vi "Get settings chain.vi"(8 "error in (no error)":errorcluster, 11 "focusBase in":refnum<class "focus.lvclass">) -> (0 "error out":errorcluster, 1 "class name":string[](array[string]), 2 "settings":variant[](array[variant]), 3 "focusBase out":refnum<class "focus.lvclass">)   [LabVIEW 2012, in "focus.lvclass"]
doc: "Returns an array of variants containing the settings clusters of each class in the inheritance chain (lowest child class first), together with an array of all class names in the inheritance chain.\n\nFor classes without settings cluster, the settings chain contains empty variants."
uses:
  focus.lvclass
  <vilib>/Distrio/Murmex/Murmex/Murmex.lvclass
  focus.lvclass/focus.ctl
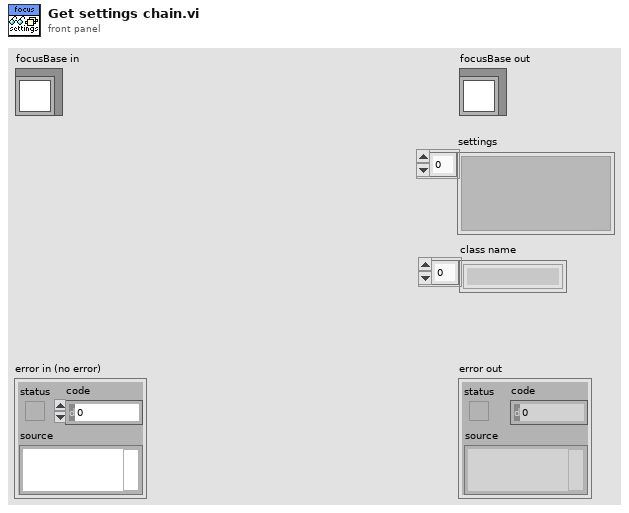
[diagram p1: front panel]
types:
  T1 = typedef "focus.lvclass/settings_cluster.ctl" = cluster{"speed":dbl[unit]}
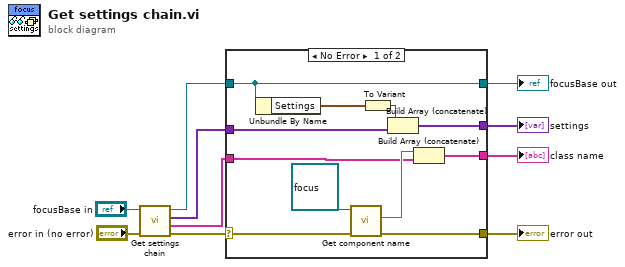
[diagram p0: block diagram]
diagram:
  n1 = call-parent "Get settings chain.vi"("error in (no error)"="error in (no error)", "MurmexBase in"="focusBase in") -> ("error out"=w8:errorcluster, "class name"=w5:string[], "settings"=w2:variant[], "MurmexBase out"=w4:refnum<class "focus.lvclass">)  [unwired: 6 in]
  n2 = case shown="No Error" w8 {
    selector: w8 -> [w20 w25]
    tunnel: [w19 w25] -> w7
    tunnel: [w16 w24] -> w6
    tunnel: w5 -> [w15 w24]
    tunnel: w4 -> [w14 w22]
    tunnel: [w14 w22] -> w3
    tunnel: w2 -> [w12 w23]
    tunnel: [w11 w23] -> w1
    frame No Error {
      n3 = Unbundle By Name(w14) -> ("Settings"=w13:T1)
      n4 = call <vilib>:"Get component name.vi"("error in (no error)"=w20, "Murmex in"=refnum<class "focus.lvclass"> refnum ("focus")) -> ("error out"=w19:errorcluster, "component name"=w17:string)  [unwired: 7 in, 1 out]
      n5 = To Variant(anything=w13) -> (Variant=w18:variant)
      n6 = Build Array (concatenate)(w18, w12) -> (w11:variant[])
      n7 = Build Array (concatenate)(w17, w15) -> (w16:string[])
    }
    frame Error {
    }
  }
  "error out" <- w7
  "focusBase out" <- w3
  "settings" <- w1
  "class name" <- w6
